vi "Send.vi"(8 "error in (no error)":errorcluster, 10 "Message":string, 11 "ILC in":refnum<class "ILC.lvclass">) -> (0 "error out":errorcluster, 3 "ILC out":refnum<class "ILC.lvclass">)   [LabVIEW 2015, in "ILCCommon.lvlib" / "ILC.lvclass"]
uses:
  <userlib>/Common/ILC/ILC/ILC.lvclass
  <userlib>/Common/ILC/ILC/ILC.lvclass/ILC.ctl
  <userlib>/Common/SerialProtocols/SerialCommunicator/SerialCommunicator.lvclass
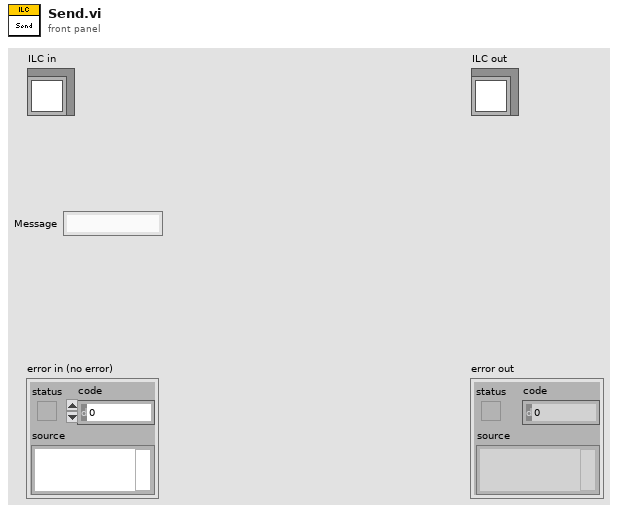
[diagram p1: front panel]
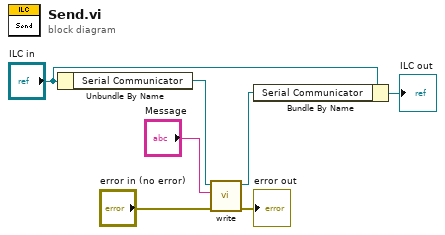
[diagram p0: block diagram]
diagram:
  n1 = Unbundle By Name("ILC in") -> ("Serial Communicator"=w6:refnum<class "SerialCommunicator.lvclass">)
  n2 = call-dynamic "write.vi"("error in (no error)"="error in (no error)", "writeString"="Message", "SerialCommunicator in"=w6) -> ("error out"=→"error out":errorcluster, "SerialCommunicator out"=w3:refnum<class "SerialCommunicator.lvclass">)  [unwired: 7 in]
  n3 = Bundle By Name(cluster="ILC in", "Serial Communicator"=w3) -> (→"ILC out":refnum<class "ILC.lvclass">)
